vi "UpdatePixelCalibrationImages.vi"(8 "Pixel Calibration Offset Image":path, 9 "Pixel Calibration Gain Image":path, 11 "Pixel calibration":T2) -> (0 "Offset":sgl[][](array[numeric]), 1 "Gain":sgl[][](array[numeric]), 3 "Pixel calibration":T2)   [LabVIEW 2011]
uses:
  Camera/PixelCalibrationDataType.ctl
  <vilib>/vision/Image Controls.llb/IMAQ Image.ctl
panel:
  out "Offset display":T1(plugin-control)
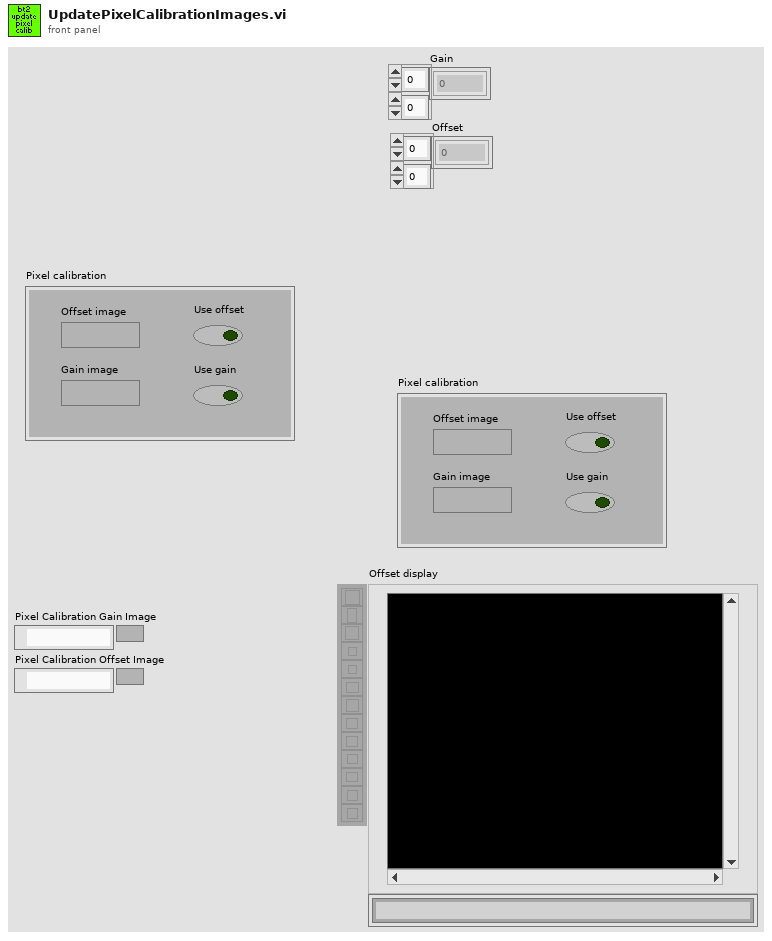
[diagram p1: front panel]
types:
  T1 = typedef "IMAQ Image.ctl" = refnum<image>
  T2 = typedef "PixelCalibrationDataType.ctl" = cluster{"Offset image":T1, "Gain image":T1, "Use offset":bool, "Use gain":bool}
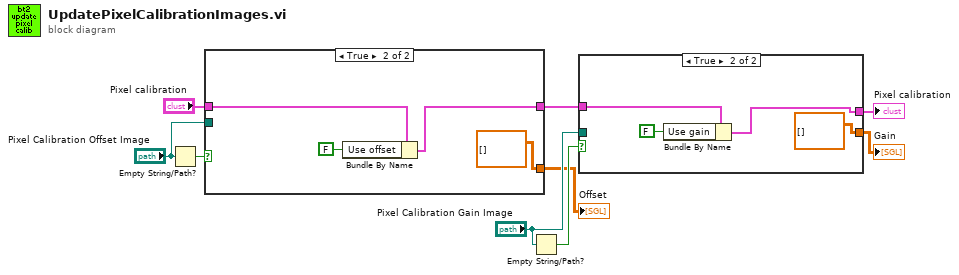
[diagram p0: block diagram]
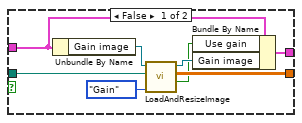
[diagram p2: hidden frame]
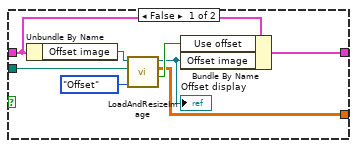
[diagram p3: hidden frame]
diagram:
  n1 = Empty String/Path?(string/path="Pixel Calibration Offset Image") -> (empty?=w7:bool)
  n2 = case shown="True" w7 {
    tunnel: "Pixel Calibration Offset Image" -> [w17 _]
    tunnel: "Pixel calibration" -> [w14 w19]
    tunnel: [w15 w18] -> w4
    tunnel: [w11 sgl[][] []] -> w1
    frame False {
      n3 = Unbundle By Name(w14) -> ("Offset image"=w16:T1)
      n4 = call "LoadAndResizeImage.vi"("Mode"=enum16{"Offset", "Gain"}."Offset", "Pixel Calibration Offset Image"=w17, "Image in"=w16) -> ("Valid"=w13:bool, "Array"=w11:sgl[][], "Image out"=w12:T1)  [unwired: 6 in]
      "Offset display" <- w12
      n5 = Bundle By Name(cluster=w14, "Use offset"=w13, "Offset image"=w12) -> (w15:T2)
    }
    frame True {
      n6 = Bundle By Name(cluster=w19, "Use offset"=FALSE) -> (w18:T2)
    }
  }
  "Offset" <- w1
  n7 = Empty String/Path?(string/path="Pixel Calibration Gain Image") -> (empty?=w6:bool)
  n8 = case shown="True" w6 {
    tunnel: "Pixel Calibration Gain Image" -> [w26 _]
    tunnel: w4 -> [w29 w32]
    tunnel: [w28 w31] -> w3
    tunnel: [w24 sgl[][] []] -> w2
    frame False {
      n9 = Unbundle By Name(w29) -> ("Gain image"=w27:T1)
      n10 = call "LoadAndResizeImage.vi"("Mode"=enum16{"Offset", "Gain"}."Gain", "Pixel Calibration Offset Image"=w26, "Image in"=w27) -> ("Valid"=w23:bool, "Array"=w24:sgl[][], "Image out"=w25:T1)  [unwired: 6 in]
      n11 = Bundle By Name(cluster=w29, "Use gain"=w23, "Gain image"=w25) -> (w28:T2)
    }
    frame True {
      n12 = Bundle By Name(cluster=w32, "Use gain"=FALSE) -> (w31:T2)
    }
  }
  "Pixel calibration" <- w3
  "Gain" <- w2
